vi "listPaths.vi"(8 "error in (no error)":errorcluster, 11 "CompiledList in":refnum<class "CompiledList.lvclass">) -> (0 "error out":errorcluster, 1 "compiledPaths":path[](array[path]), 2 "Array":path[](array[path]), 3 "CompiledList out":refnum<class "CompiledList.lvclass">)   [LabVIEW 2011, in "Compiler.lvlib" / "CompiledList.lvclass"]
uses:
  CompiledList.lvclass
  CompiledList.lvclass/CompiledList.ctl
  ScriptListCompiler/ScriptListCompiler.lvclass
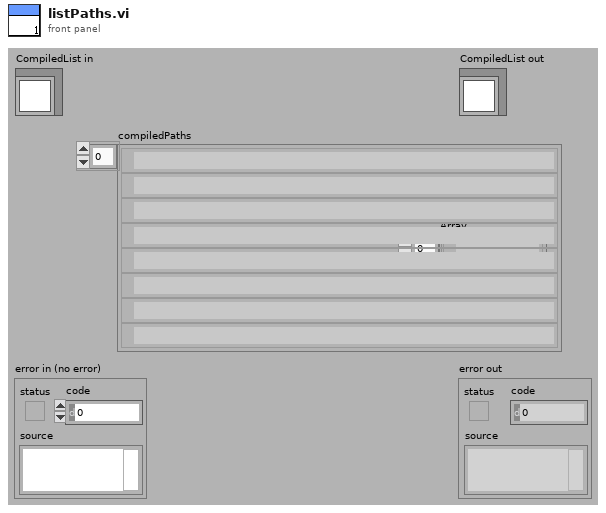
[diagram p1: front panel]
types:
  T1 = cluster{"ScriptListCompiler.lvclass":refnum<class "ScriptListCompiler.lvclass">, "aoChannels":refnum<class "AnalogOutput.lvclass">[], "doChannels":refnum<class "DigitalOutput.lvclass">[], "rfChannels":refnum<class "DDSOutput.lvclass">[]}[]
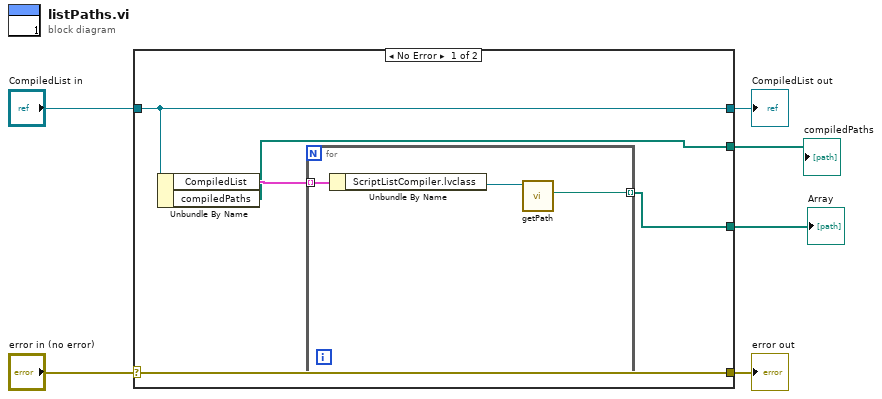
[diagram p0: block diagram]
diagram:
  n1 = case shown="No Error" "error in (no error)" {
    selector: "error in (no error)" -> [w11 w16]
    tunnel: [w11 w16] -> w5
    tunnel: [w10 w15] -> w3
    tunnel: "CompiledList in" -> [w10 w15]
    tunnel: [w8 _] -> w2
    tunnel: [w7 _] -> w1
    frame No Error {
      n2 = Unbundle By Name(w10) -> ("CompiledList"=w9:T1, "compiledPaths"=w7:path[])
      n3 = for {
        tunnel: w9 -> [w14] mode=indexing
        tunnel: [w12] -> w8 mode=indexing
        n4 = Unbundle By Name(w14) -> ("ScriptListCompiler.lvclass"=w13:refnum<class "ScriptListCompiler.lvclass">)
        n5 = call "getPath.vi"("ScriptListCompiler in"=w13) -> ("Path"=w12:path)  [unwired: 8 in, 2 out]
      }
    }
    frame Error {
    }
  }
  "error out" <- w5
  "CompiledList out" <- w3
  "Array" <- w2
  "compiledPaths" <- w1
